vi "JSON_extract_Type (SubVI).vi"(11 "data in":string) -> (0 "id":i32, 2 "Type":string)   [LabVIEW 2015]
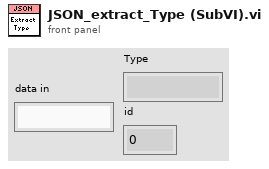
[diagram p1: front panel]
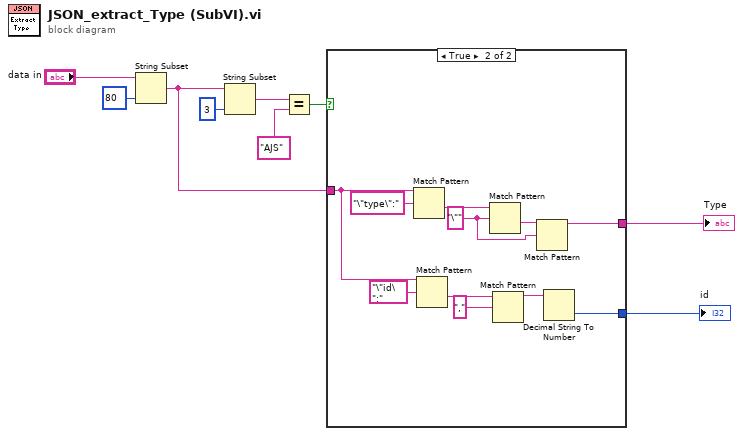
[diagram p0: block diagram]
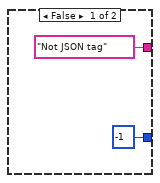
[diagram p2: hidden frame]
diagram:
  n1 = String Subset(string="data in", length (rest)=80 ("length (rest)")) -> (substring=w3:string)  [unwired: 1 in]
  n2 = String Subset(string=w3, length (rest)=3 ("length (rest)")) -> (substring=w6:string)  [unwired: 1 in]
  n3 = Equal?(x=w6, y="AJS") -> (x = y?=w4:bool)
  n4 = case shown="True" w4 {
    tunnel: w3 -> [_ w14]
    tunnel: ["Not JSON tag" ("data in") w18] -> w2
    tunnel: [-1 w12] -> w1
    frame False {
    }
    frame True {
      w19 = "\"" ("regular expression")
      n5 = Match Pattern(string=w14, regular expression="\"type\":") -> (after substring=w21:string)  [unwired: 1 in, 3 out]
      n6 = Match Pattern(string=w14, regular expression="\"id\":") -> (after substring=w16:string)  [unwired: 1 in, 3 out]
      n7 = Match Pattern(string=w21, regular expression=w19) -> (after substring=w20:string)  [unwired: 1 in, 3 out]
      n8 = Match Pattern(string=w16, regular expression=",") -> (before substring=w13:string)  [unwired: 1 in, 3 out]
      n9 = Match Pattern(string=w20, regular expression=w19) -> (before substring=w18:string)  [unwired: 1 in, 3 out]
      n10 = Decimal String To Number(string=w13) -> (number=w12:i32)  [unwired: 2 in, 1 out]
    }
  }
  "Type" <- w2
  "id" <- w1
